vi "Timer2.vi"() -> ()   [LabVIEW 2015]
panel:
  in  "stop":bool
  out "Elapsed Time":dbl
  out "Llegada":bool
  in  "Delay":dbl
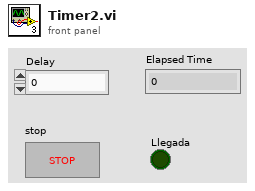
[diagram p1: front panel]
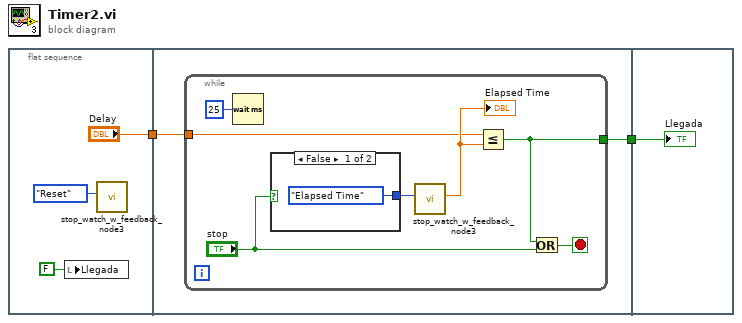
[diagram p0: block diagram]
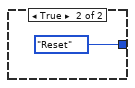
[diagram p2: hidden frame]
diagram:
  n1 = flat-sequence {
    tunnel: ["Delay"] -> w2
    tunnel: w2 -> [w7]
    tunnel: [w6] -> w1
    tunnel: w1 -> [w17]
    frame #0 {
      n2 = local write "Llegada"(FALSE ("Boolean")) -> ()
      n3 = call "stop_watch_w_feedback_node3.vi"("Command"=enum16{"Elapsed Time", "Reset"}."Reset") -> ()  [unwired: 10 in, 1 out]
    }
    frame #1 {
      n4 = while {
        tunnel: w7 -> [w13]
        tunnel: [w10] -> w6
        stop <- w9 stop-if-true
        n5 = Wait (ms)(milliseconds to wait=u32 25) -> ()  [unwired: 1 out]
        n6 = case shown="False" "stop" {
          tunnel: [enum16{"Elapsed Time", "Reset"}."Elapsed Time" ("Command") enum16{"Elapsed Time", "Reset"}."Reset" ("Command")] -> w12
          frame False {
          }
          frame True {
          }
        }
        n7 = call "stop_watch_w_feedback_node3.vi"("Command"=w12) -> ("Elapsed Time"=w14:dbl)  [unwired: 10 in]
        "Elapsed Time" <- w14
        n8 = Less Or Equal?(x=w13, y=w14) -> (x <= y?=w10:bool)
        n9 = Or(x=w10, y="stop") -> (x .or. y?=w9:bool)
      }
    }
    frame #2 {
      "Llegada" <- w17
    }
  }
